vi "OnValueChange_rightJoy.vi"(8 "error in (no error)":errorcluster, 9 "direction":T1, 10 "Engine":refnum<class "Engine.lvclass">, 11 "Game in":refnum<class "Game.lvclass">) -> (0 "error out":errorcluster, 2 "Engine out":refnum<class "Engine.lvclass">, 3 "Game out":refnum<class "Game.lvclass">)   [LabVIEW 2019, in "RT_Game.lvlib" / "Game.lvclass"]
uses:
  Game.lvclass
  Engine/Engine.lvclass
  Engine/JoystickDir.ctl
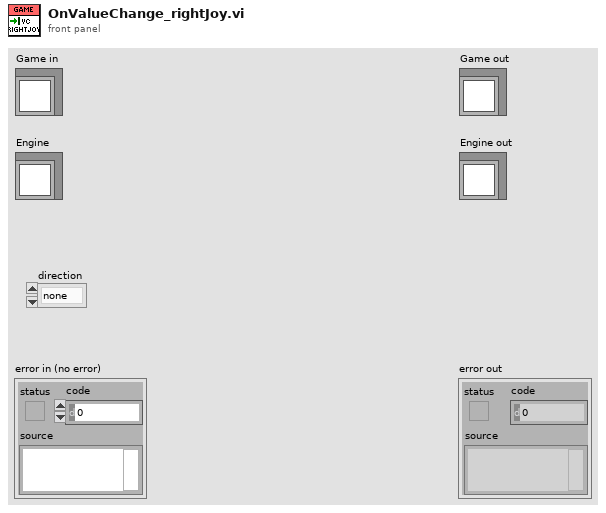
[diagram p1: front panel]
types:
  T1 = typedef "RT_Game.lvlib/Engine.lvclass/JoystickDir.ctl" = enum16{"none", "left", "right", "leftrightUNUSED", "up", "upLeft", "upRight", "upLeftRightUNUSED", "down", "downLeft", "downRight", "downLeftRightUNUSED", "upDownUNUSED", "upDownLeftUNUSED", "upDownRightUNUSED", "upDownRightLeftUNUSED"}
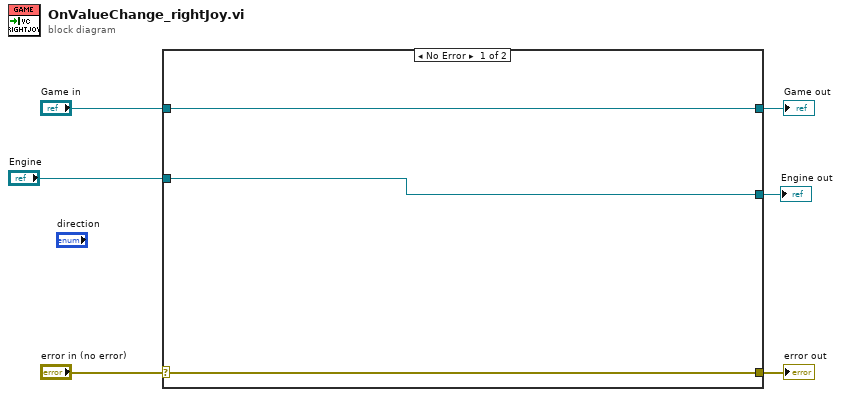
[diagram p0: block diagram]
diagram:
  n1 = case shown="No Error" "error in (no error)" {
    selector: "error in (no error)" -> [w8 w12]
    tunnel: [w8 w12] -> w5
    tunnel: [w9 w11] -> w3
    tunnel: "Game in" -> [w9 w11]
    tunnel: "Engine" -> [w7 w10]
    tunnel: [w7 w10] -> w1
    frame No Error {
    }
    frame Error {
    }
  }
  "error out" <- w5
  "Game out" <- w3
  "Engine out" <- w1
